vi "CE14. Read_PowerFactor(subVI).vi"(8 "error in (no error)":errorcluster, 9 "milliseconds to wait(200)":u32=200, 11 "VISA resource name":refnum<visa-resource-name>) -> (0 "error out":errorcluster, 1 "data out":T1, 2 "read buffer":string, 3 "VISA resource name out":refnum<visa-resource-name>)   [LabVIEW 2018, in "CE14_eMIC.lvlib"]
uses:
  CE14_eMIC.lvlib
  type defs/CE14.data.ctl
  <vilib>/Instr/_visa.llb/VISA Flush IO Buffer Mask.ctl
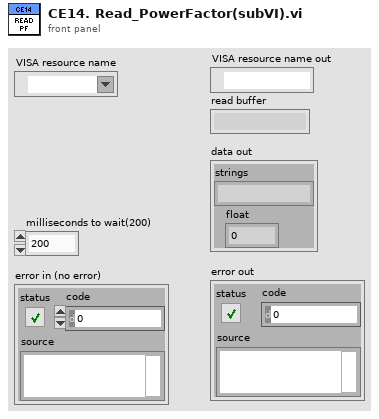
[diagram p1: front panel]
types:
  T1 = typedef "CE14_eMIC.lvlib/CE14.data.ctl" = cluster{"strings":string, "float":dbl}
  T2 = typedef "VISA Flush IO Buffer Mask.ctl" = u16
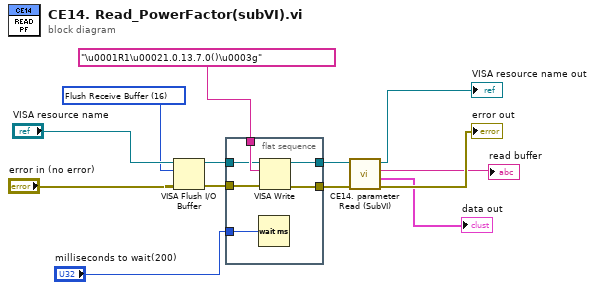
[diagram p0: block diagram]
diagram:
  w5 = T2 16 items=["Flush Receive Buffer"=16, "Write Transmit Buffer to Device"=32, "Flush Receive Buffer (No I/O)"=64, "Flush Transmit Buffer"=128] ("Mask")
  n1 = VISA Flush I/O Buffer(VISA resource name="VISA resource name", mask (16)=w5, error in (no error)="error in (no error)") -> (VISA resource name out=w8:refnum<visa-resource-name>, error out=w9:errorcluster)
  n2 = flat-sequence {
    tunnel: "\u0001R1\u00021.0.13.7.0()\u0003g" -> [w19]
    tunnel: w8 -> [w18]
    tunnel: w9 -> [w17]
    tunnel: [w16] -> w12
    tunnel: [w15] -> w11
    tunnel: "milliseconds to wait(200)" -> [w14]
    frame #0 {
      n3 = Wait (ms)(milliseconds to wait=w14) -> ()  [unwired: 1 out]
      n4 = VISA Write(VISA resource name=w18, write buffer=w19, error in (no error)=w17) -> (VISA resource name out=w15:refnum<visa-resource-name>, error out=w16:errorcluster)  [unwired: 1 out]
    }
  }
  n5 = call "CE14. parameter Read (SubVI).vi"("error in (no error)"=w12, "VISA Refnum in"=w11) -> ("error out"=→"error out":errorcluster, "data out"=→"data out":T1, "read buffer"=→"read buffer":string, "VISA Refnum out"=→"VISA resource name out":refnum<visa-resource-name>)  [unwired: 4 in, 2 out]
